vi "Calc Bottom To Mid Deltas.vi"(7 "Texture Dimensions":T2, 11 "UVs":cluster{"Top":T1, "Middle":T1, "Bottom":T1} {"Bottom"."v" min=0 max=1 step=0.1; "Bottom"."u" min=0 max=1 step=0.1; "Middle"."v" min=0 max=1 step=0.1; "Middle"."u" min=0 max=1 step=0.1; "Top"."v" min=0 max=1 step=0.1; "Top"."u" min=0 max=1 step=0.1}) -> (3 "Deltas (Pixels)":T1 {"v" min=0 max=1 step=0.1; "u" min=0 max=1 step=0.1})   [LabVIEW 2022 SP3]
uses:
  Raster.lvlib
  UV.ctl
  Rectangle Dimensions.ctl
panel:
  in  "Start Position":T1={"u"=0.3019608, "v"=-2.2313726} {"v" min=0 max=1 step=0.1; "u" min=0 max=1 step=0.1}
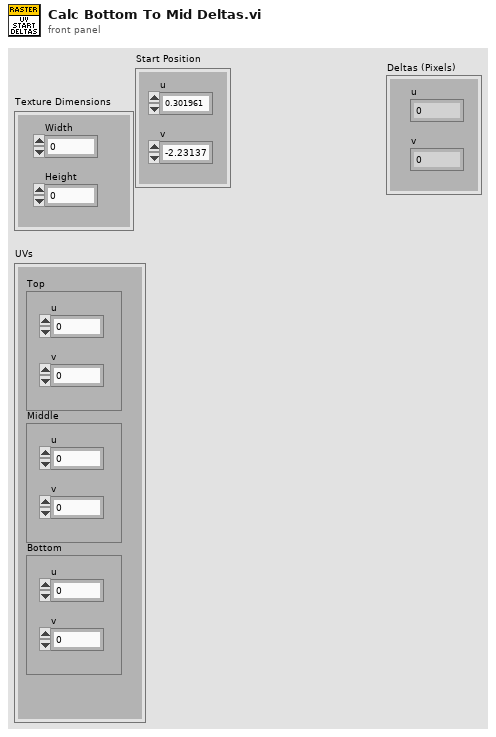
[diagram p1: front panel]
types:
  T1 = typedef "Raster.lvlib/UV.ctl" = cluster{"u":sgl, "v":sgl}
  T2 = typedef "Raster.lvlib/Rectangle Dimensions.ctl" = cluster{"Width":u32, "Height":u32}
  T3 = typedef "Raster.lvlib/Line Parameters.ctl" = cluster{"1/m":sgl, "c":sgl}
  T4 = typedef "Raster.lvlib/Point 2D.ctl" = cluster{"x":i32, "y":i32}
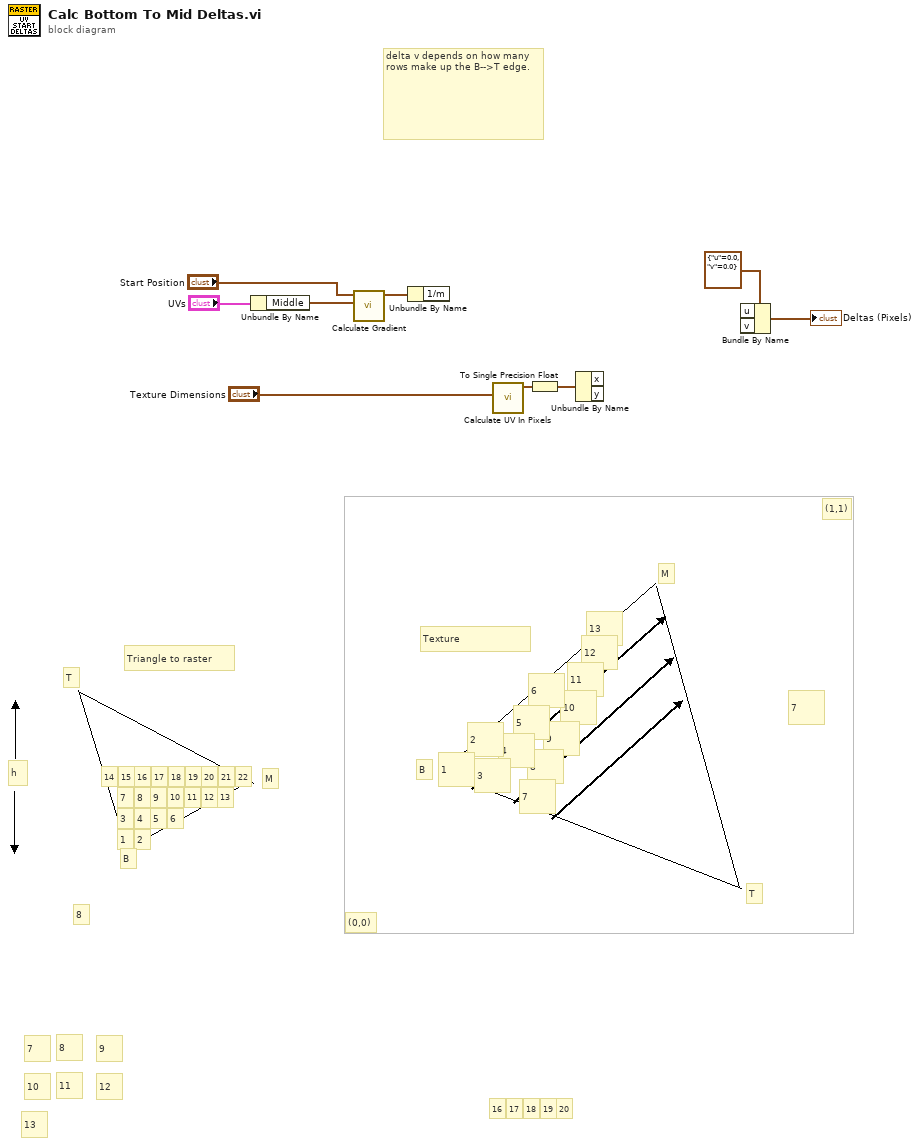
[diagram p0: block diagram]
diagram:
  # "13"
  # "12"
  # "11"
  # "10"
  # "9"
  # "8"
  # "7"
  # "7"
  # "6"
  # "5"
  # "4"
  # "3"
  # "2"
  # "20"
  # "19"
  # "18"
  # "17"
  # "16"
  # "15"
  # "14"
  # "20"
  # "19"
  # "18"
  # "17"
  # "16"
  # "22"
  # "21"
  # "8"
  # "13"
  # "12"
  # "11"
  # "10"
  # "9"
  # "8"
  # "7"
  # "1"
  # "13"
  # "12"
  # "11"
  # "10"
  # "9"
  # "8"
  # "7"
  # "6"
  # "5"
  # "4"
  # "3"
  # "2"
  # "1"
  # "(0,0)"
  # "(1,1)"
  # "h"
  # "Texture"
  # "Triangle to raster"
  # "M"
  # "T"
  # "B"
  # "delta v depends on how many rows make up the B-->T edge."
  # "T"
  # "M"
  # "B"
  n1 = Unbundle By Name("UVs") -> ("Middle"=w3:T1)
  n2 = call "Calculate Gradient.vi"("P2"=w3, "P1"="Start Position") -> ("Line Parameters"=w5:T3)  [unwired: 9 in]
  n3 = Unbundle By Name(w5) -> ()  [unwired: 1 out]
  n4 = call "Calculate UV In Pixels.vi"(10:"Texture Dimensions") -> ("Pixels"=w9:T4)  [unwired: 10 in]
  n5 = To Single Precision Float(number=w9) -> (single precision float=w8:cluster{"x":sgl, "y":sgl})
  n6 = Unbundle By Name(w8) -> ()  [unwired: 2 out]
  n7 = Bundle By Name(cluster=T1 {"u"=0.0, "v"=0.0} ("Start Deltas")) -> (→"Deltas (Pixels)":T1, "u"=w7:sgl, "v"=w6:sgl)
